vi "PPR_TRAJ_Creation_Abs.vi"(8 "End Pose  ENG":T15={"TRANSLATION"={"X"=0.0, "Y"=0.0}, "ROTATION"={"VALUE"=0.0, "COS"=1.0, "SIN"=0.0}} {"ROTATION"."SIN" format="%13.4f"; "ROTATION"."COS" format="%13.4f"; "ROTATION"."VALUE" format="%13.4f"; "TRANSLATION"."Y" format="%14.3f"; "TRANSLATION"."X" format="%14.3f"}, 9 "Current Pose SI":T15={"TRANSLATION"={"X"=0.0, "Y"=0.0}, "ROTATION"={"VALUE"=0.0, "COS"=1.0, "SIN"=0.0}} {"ROTATION"."SIN" format="%13.4f"; "ROTATION"."COS" format="%13.4f"; "ROTATION"."VALUE" format="%13.4f"; "TRANSLATION"."Y" format="%14.3f"; "TRANSLATION"."X" format="%14.3f"}, 10 "Max Velocity M/S":dbl=2.3 format="%17.3f") -> (0 "Path\nCreation\nError":bool, 1 "PathPlannerTrajectory":T16 {"States"."TargetHolonomicRotation"."SIN" format="%13.4f"; "States"."TargetHolonomicRotation"."COS" format="%13.4f"; "States"."TargetHolonomicRotation"."VALUE" format="%13.4f"; "States"."Heading"."SIN" format="%13.4f"; "States"."Heading"."COS" format="%13.4f"; "States"."Heading"."VALUE" format="%13.4f"; "States"."PositionMeters"."Y" format="%14.3f"; "States"."PositionMeters"."X" format="%14.3f"}, 3 "TotalTImeSecs":dbl)   [LabVIEW 2019]
uses:
  <vilib>/Rock Robotics/WPI/ThirdParty/JAS_Junk/TrajLib/Trajectory_Library.lvlib
  <vilib>/Rock Robotics/WPI/ThirdParty/MJansen/PathPlanner/PathPlanner24.lvlib
  <vilib>/Rock Robotics/WPI/ThirdParty/JAS_Junk/TrajLib/TypeDef/TRANSLATION2D.ctl
  <vilib>/Rock Robotics/WPI/ThirdParty/JAS_Junk/TrajLib/TypeDef/ROTATION2D.ctl
  <vilib>/Rock Robotics/WPI/ThirdParty/MJansen/PathPlanner/TypeDef/PathPlannerPathConstraints.ctl
  <vilib>/Rock Robotics/WPI/ThirdParty/MJansen/PathPlanner/TypeDef/PathPlannerTrajectoryState.ctl
  <vilib>/Rock Robotics/WPI/ThirdParty/MJansen/PathPlanner/TypeDef/PathPlannerTrajectory.ctl
  <vilib>/Rock Robotics/WPI/ThirdParty/JAS_Junk/TrajLib/TypeDef/POSE2D.ctl
  <vilib>/Rock Robotics/WPI/ThirdParty/MJansen/PathPlanner/TypeDef/PathPlannerRotationTarget.ctl
  <vilib>/Rock Robotics/WPI/ThirdParty/MJansen/PathPlanner/TypeDef/PathPlannerConstraintsZone.ctl
  <vilib>/Rock Robotics/WPI/ThirdParty/MJansen/PathPlanner/ENum/PathPlanner_CommandUtilType_ENUM.ctl
  <vilib>/Rock Robotics/WPI/ThirdParty/MJansen/PathPlanner/TypeDef/PathPlannerCommandUtil.ctl
  <vilib>/Rock Robotics/WPI/ThirdParty/MJansen/PathPlanner/TypeDef/PathPlannerEventMarker.ctl
  <vilib>/Rock Robotics/WPI/ThirdParty/MJansen/PathPlanner/TypeDef/PathPlannerGoalEndState.ctl
  <vilib>/Rock Robotics/WPI/ThirdParty/MJansen/PathPlanner/TypeDef/PathPlannerPathPoint.ctl
  <vilib>/Rock Robotics/WPI/ThirdParty/MJansen/PathPlanner/TypeDef/PathPlannerPath.ctl
  <vilib>/Rock Robotics/WPI/ThirdParty/MJansen/PathPlanner/TypeDef/PathPlannerWaypoint.ctl
  <vilib>/Rock Robotics/WPI/ThirdParty/MJansen/PathPlanner/TypeDef/PathPlannerPointTowardsZone.ctl
  <vilib>/Rock Robotics/WPI/ThirdParty/MJansen/PathPlanner/TypeDef/PathPlannerIdealStartingState.ctl
panel:
  out "PathPlannerPath":T1={"Reversed"=FALSE, "RotationTargets"=[], "ConstraintZones"=[], "EventMarkers"=[], "GlobalConstraints"={"MaxVelocityMps;"=0.0, "MaxAccelerationMpsSq;"=0.0, "MaxAngularVelRadPsEc;"=0.0, "MaxAngularAccRadPSecSq"=0.0, "Exists"=FALSE, "Unlimited"=FALSE, "NominalVoltageVolts"=1.0}, "GoalEndState"={"VelocityMPS"=0.0, "Rotation"={"VALUE"=0.0, "COS"=1.0, "SIN"=0.0}}, "AllPoints"=[], "Name"="", "Waypoints"=[], "PointTowardsZones"=[], "IdealStartingState"={"VelocityMPS"=0.0, "Rotation"={"VALUE"=0.0, "COS"=1.0, "SIN"=0.0}}, "IsChoreoPath"=FALSE, "PreventFlipping"=FALSE} {"IdealStartingState"."Rotation"."SIN" format="%13.4f"; "IdealStartingState"."Rotation"."COS" format="%13.4f"; "IdealStartingState"."Rotation"."VALUE" format="%13.4f"; "PointTowardsZones"."TargetPosition"."Y" format="%14.3f"; "PointTowardsZones"."TargetPosition"."X" format="%14.3f"; "PointTowardsZones"."RotationOffset"."SIN" format="%13.4f"; "PointTowardsZones"."RotationOffset"."COS" format="%13.4f"; "PointTowardsZones"."RotationOffset"."VALUE" format="%13.4f"; "Waypoints"."nextControl"."Y" format="%14.3f"; "Waypoints"."nextControl"."X" format="%14.3f"; "Waypoints"."anchor"."Y" format="%14.3f"; "Waypoints"."anchor"."X" format="%14.3f"; "Waypoints"."prevControl"."Y" format="%14.3f"; "Waypoints"."prevControl"."X" format="%14.3f"; "AllPoints"."RotationTarget"."rotation"."SIN" format="%13.4f"; "AllPoints"."RotationTarget"."rotation"."COS" format="%13.4f"; "AllPoints"."RotationTarget"."rotation"."VALUE" format="%13.4f"; "AllPoints"."Position"."Y" format="%14.3f"; "AllPoints"."Position"."X" format="%14.3f"; "GoalEndState"."Rotation"."SIN" format="%13.4f"; "GoalEndState"."Rotation"."COS" format="%13.4f"; "GoalEndState"."Rotation"."VALUE" format="%13.4f"; "RotationTargets"."rotation"."SIN" format="%13.4f"; "RotationTargets"."rotation"."COS" format="%13.4f"; "RotationTargets"."rotation"."VALUE" format="%13.4f"}
  in  "End Velocity M/S":dbl format="%#_13g"
  in  "Start Angual Vel Rad/S":dbl format="%#_13g"
  in  "Start Y Vel M/S":dbl format="%#_13g"
  in  "Start X Vel M/S":dbl format="%#_13g"
  in  "MaxAngularAccel Radians.Sec^2":dbl=1.0 format="%17.3f"
  out "Trajectory":cluster{dbl[], dbl[]}(graph)
  out "Trajectory State\nCount":i32
  in  "MaxAcceleration M/S^2":dbl=1.6 format="%17.1f"
  in  "MaxAngularVel  Radians/Sec":dbl=1.5 format="%17.3f"
  # "Create PathPlanner Path/Trajectory Sample"
  # "This VI is designed to be called by BEGIN.VI, but can be executed directly to test trajectory parameters."
  # "CREATED TRAJECTORY INFORMATION"
  # "PATH CONFIGURATION"
  # "PATH DEFINITION"
  # "There can be as many points as needed."
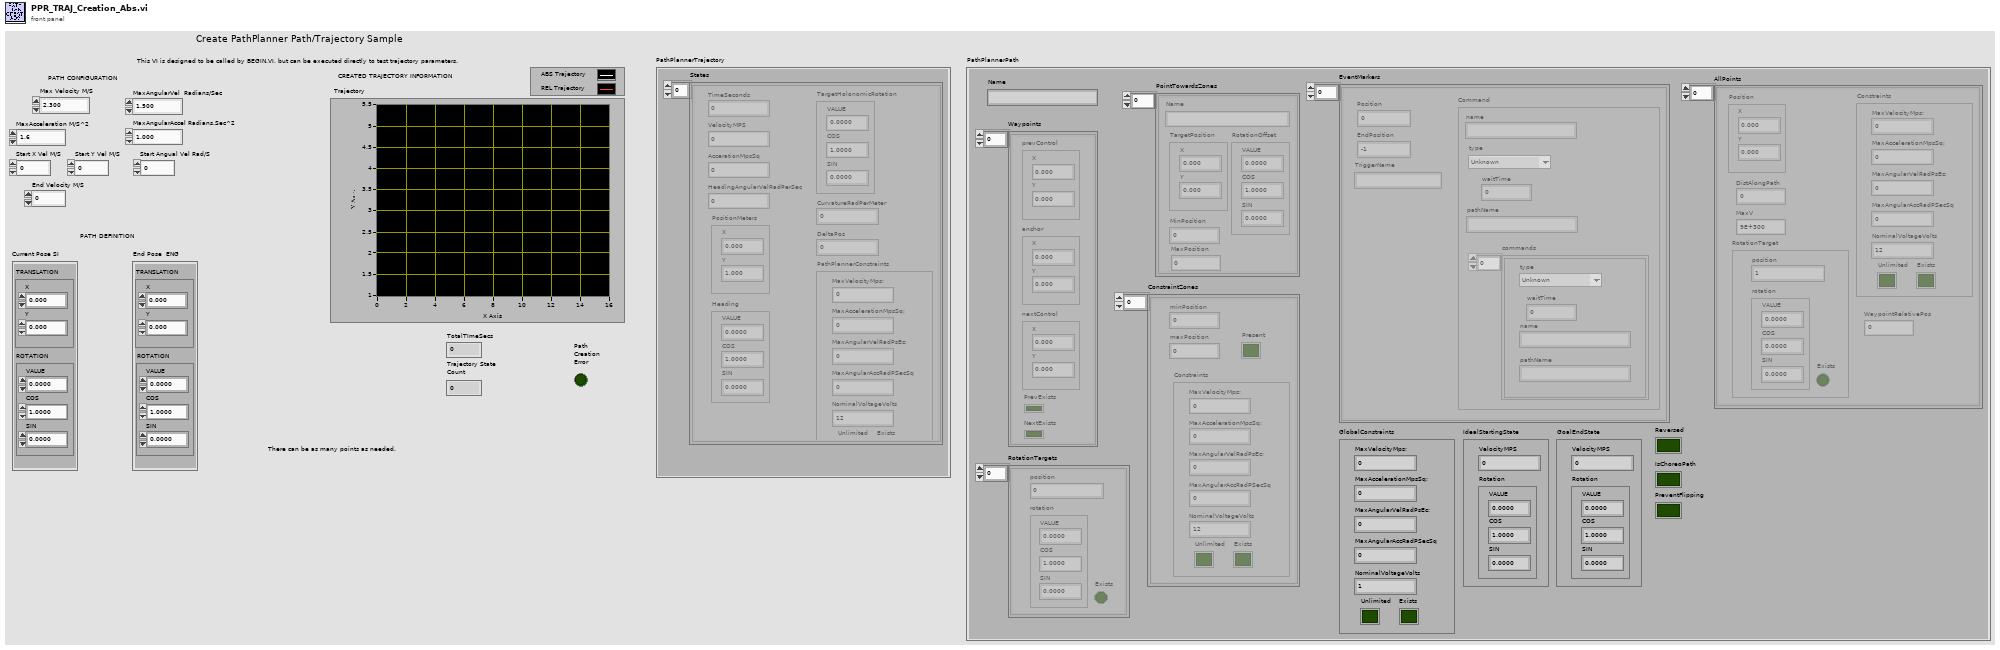
[diagram p1: front panel]
types:
  T1 = typedef "PathPlanner24.lvlib/PathPlannerPath.ctl" = cluster{"Reversed":bool, "RotationTargets":T2[], "ConstraintZones":T4[], "EventMarkers":T6[], "GlobalConstraints":T5, "GoalEndState":T9, "AllPoints":T10[], "Name":string, "Waypoints":T12[], "PointTowardsZones":T13[], "IdealStartingState":T14, "IsChoreoPath":bool, "PreventFlipping":bool}
  T2 = typedef "PathPlanner24.lvlib/PathPlannerRotationTarget.ctl" = cluster{"position":dbl, "rotation":T3, "Exists":bool}
  T3 = typedef "Trajectory_Library.lvlib/ROTATION2D.ctl" = cluster{"VALUE":dbl, "COS":dbl, "SIN":dbl}
  T4 = typedef "PathPlanner24.lvlib/PathPlannerConstraintsZone.ctl" = cluster{"minPosition":dbl, "maxPosition":dbl, "Constraints":T5, "Present":bool}
  T5 = typedef "PathPlanner24.lvlib/PathPlannerPathConstraints.ctl" = cluster{"MaxVelocityMps;":dbl, "MaxAccelerationMpsSq;":dbl, "MaxAngularVelRadPsEc;":dbl, "MaxAngularAccRadPSecSq":dbl, "Exists":bool, "Unlimited":bool, "NominalVoltageVolts":dbl}
  T6 = typedef "PathPlanner24.lvlib/PathPlannerEventMarker.ctl" = cluster{"Position":dbl, "Command":T7, "TriggerName":string, "EndPosition":dbl}
  T7 = typedef "PathPlanner24.lvlib/PathPlannerCommandUtil.ctl" = cluster{"waitTime":dbl, "name":string, "pathName":string, "commands":cluster{"type":T8, "waitTime":dbl, "name":string, "pathName":string}[], "type":T8}
  T8 = typedef "PathPlanner24.lvlib/PathPlanner_CommandUtilType_ENUM.ctl" = enum16{"Unknown", "Wait", "Named", "Path", "Sequential", "Parallel", "Race", "Deadline"}
  T9 = typedef "PathPlanner24.lvlib/PathPlannerGoalEndState.ctl" = cluster{"VelocityMPS":dbl, "Rotation":T3}
  T10 = typedef "PathPlanner24.lvlib/PathPlannerPathPoint.ctl" = cluster{"Position":T11, "DistAlongPath":dbl, "MaxV":dbl, "Constraints":T5, "RotationTarget":T2, "WaypointRelativePos":dbl}
  T11 = typedef "Trajectory_Library.lvlib/TRANSLATION2D.ctl" = cluster{"X":dbl, "Y":dbl}
  T12 = typedef "PathPlanner24.lvlib/PathPlannerWaypoint.ctl" = cluster{"prevControl":T11, "anchor":T11, "nextControl":T11, "PrevExists":bool, "NextExists":bool}
  T13 = typedef "PathPlanner24.lvlib/PathPlannerPointTowardsZone.ctl" = cluster{"RotationOffset":T3, "Name":string, "TargetPosition":T11, "MinPosition":dbl, "MaxPosition":dbl}
  T14 = typedef "PathPlanner24.lvlib/PathPlannerIdealStartingState.ctl" = cluster{"VelocityMPS":dbl, "Rotation":T3}
  T15 = typedef "Trajectory_Library.lvlib/POSE2D.ctl" = cluster{"TRANSLATION":T11, "ROTATION":T3}
  T16 = typedef "PathPlanner24.lvlib/PathPlannerTrajectory.ctl" = cluster{"States":T17[]}
  T17 = typedef "PathPlanner24.lvlib/PathPlannerTrajectoryState.ctl" = cluster{"TimeSeconds":dbl, "VelocityMPS":dbl, "AccerationMpsSq":dbl, "HeadingAngularVelRadPerSec":dbl, "PositionMeters":T11, "Heading":T3, "TargetHolonomicRotation":T3, "CurvatureRadPerMeter":dbl, "PathPlannerConstraints":T5, "DeltaPos":dbl}
  T18 = typedef "Trajectory_Library.lvlib/CHASSIS_SPEEDS.ctl" = cluster{"vX":dbl, "vY":dbl, "vOmega":dbl}
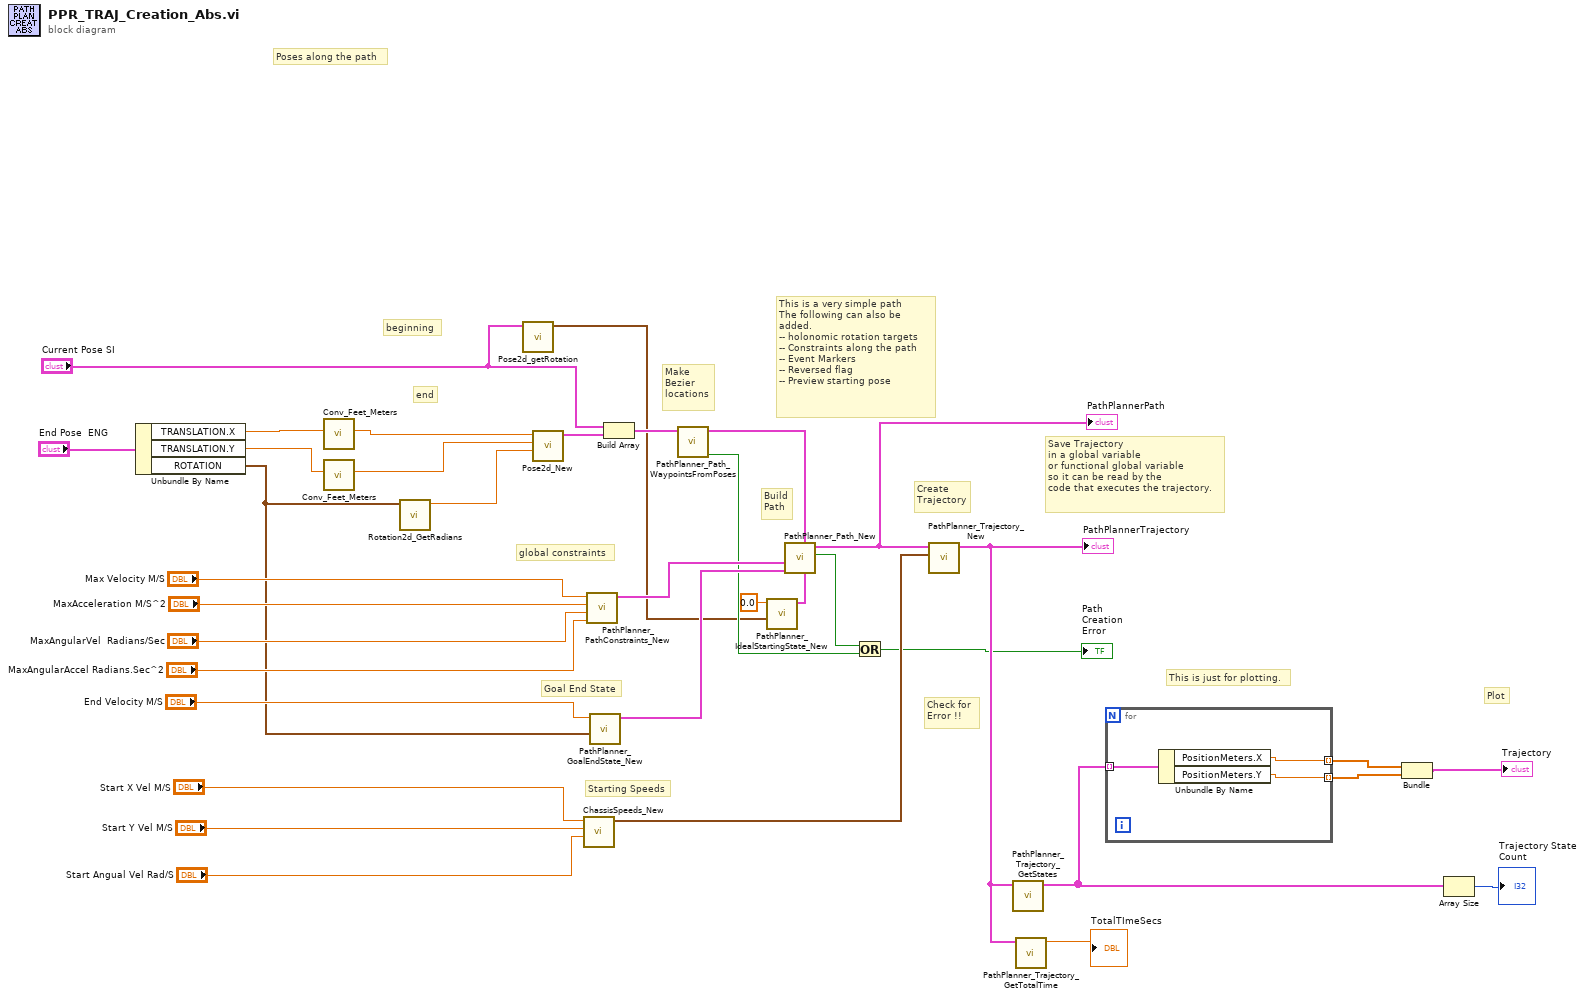
[diagram p0: block diagram]
diagram:
  # "This is just for plotting."
  # "end"
  # "beginning"
  # "This is a very simple path\nThe following can also be\nadded.\n-- holonomic rotation targets\n-- Constraints along the path\n-- Event Markers\n-- Reversed flag\n-- Preview starting pose"
  # "Plot"
  # "Save Trajectory\nin a global variable\nor functional global variable\nso it can be read by the \ncode that executes the trajectory."
  # "Create\nTrajectory"
  # "Check for\nError !!"
  # "Starting Speeds"
  # "Goal End State"
  # "global constraints"
  # "Make\nBezier\nlocations"
  # "Build\nPath"
  # "Poses along the path"
  n1 = Unbundle By Name("End Pose  ENG") -> ("TRANSLATION.X"=w15:dbl, "TRANSLATION.Y"=w14:dbl, "ROTATION"=w8:T3)
  n2 = call <vilib>:"Conv_Feet_Meters.vi"("Feet"=w15) -> ("Meters"=w10:dbl)  [unwired: 10 in]
  n3 = call <vilib>:"Conv_Feet_Meters.vi"("Feet"=w14) -> ("Meters"=w9:dbl)  [unwired: 10 in]
  n4 = call <vilib>:"Rotation2d_GetRadians.vi"("in ROTATION"=w8) -> ("AngleRadians"=w7:dbl)  [unwired: 10 in]
  n5 = call <vilib>:"Pose2d_getRotation.vi"("in POSE"="Current Pose SI") -> ("out ROTATION"=w2:T3)  [unwired: 10 in]
  n6 = call <vilib>:"Pose2d_New.vi"("Heading"=w7, "Y"=w9, "X"=w10) -> ("out POSe"=w6:T15)  [unwired: 8 in]
  n7 = call <vilib>:"ChassisSpeeds_New.vi"("vAngular"="Start Angual Vel Rad/S", "vY"="Start Y Vel M/S", "vX"="Start X Vel M/S") -> ("CHASSIS"=w35:T18)  [unwired: 8 in]
  n8 = call <vilib>:"PathPlanner_PathConstraints_New.vi"("MaxAngularAccRadPSecSq"="MaxAngularAccel Radians.Sec^2", "MaxAngularVelRadPsEc;"="MaxAngularVel  Radians/Sec", "MaxAccelerationMpsSq;"="MaxAcceleration M/S^2", "MaxVelocityMps;"="Max Velocity M/S") -> ("PathPlannerConstraints"=w28:T5)  [unwired: 7 in]
  n9 = call <vilib>:"PathPlanner_GoalEndState_New.vi"("Rotation"=w8, "VelocityMPS"="End Velocity M/S") -> ("GoalEndState"=w30:T9)  [unwired: 9 in]
  n10 = Build Array("Current Pose SI", w6) -> (w26:T15[])
  n11 = call <vilib>:"PathPlanner_Path_WaypointsFromPoses.vi"("Poses"=w26) -> ("Error"=w11:bool, "Waypoints"=w27:T12[])  [unwired: 9 in]
  n12 = call <vilib>:"PathPlanner_IdealStartingState_New.vi"("Rotation"=w2, "VelocityMPS"=0.0) -> ("IdealStartingState"=w1:T14)  [unwired: 9 in]
  n13 = call <vilib>:"PathPlanner_Path_New.vi"("IdealStartingState"=w1, "Waypoints"=w27, "GoalEndState"=w30, "GlobalConstraints"=w28) -> ("Error"=w5:bool, "PathPlannerPath"=w31:T1)  [unwired: 6 in]
  "PathPlannerPath" <- w31
  n14 = Or(x=w5, y=w11) -> (x .or. y?=→"Path\nCreation\nError":bool)
  n15 = call <vilib>:"PathPlanner_Trajectory_New.vi"("StartingSpeeds"=w35, "Path"=w31) -> ("PathPlannerTrajectory"=w21:T16)  [unwired: 8 in, 1 out]
  "PathPlannerTrajectory" <- w21
  n16 = call <vilib>:"PathPlanner_Trajectory_GetStates.vi"("PathPlannerTrajectory"=w21) -> ("PathPlannerStates"=w22:T17[])  [unwired: 10 in]
  n17 = call <vilib>:"PathPlanner_Trajectory_GetTotalTime.vi"("PathPlannerTrajectory"=w21) -> ("TotalTimeSeconds"=→"TotalTImeSecs":dbl)  [unwired: 10 in]
  n18 = for {
    tunnel: [w39] -> w24 mode=indexing
    tunnel: [w38] -> w25 mode=indexing
    tunnel: w22 -> [w37] mode=indexing
    n19 = Unbundle By Name(w37) -> ("PositionMeters.X"=w39:dbl, "PositionMeters.Y"=w38:dbl)
  }
  n20 = Bundle(w24, w25) -> (→"Trajectory":cluster{dbl[], dbl[]})  [unwired: 1 in]
  n21 = Array Size(array=w22) -> (size(s)=→"Trajectory State\nCount":i32)
